vi "GL_SamplerateDispl.vi"() -> ()   [LabVIEW 2019]
panel:
  out "SAMPLE RATE":dbl=1.0 min=0.0 max=600.0 step=0.001 format="%.3f"
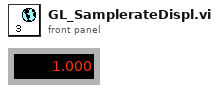
[diagram p1: front panel]
diagram:
